vi "TCP Engine Get Msg From Host.vi"(8 "error in (no error)":errorcluster, 11 "Data Cluster in":T1 {"Hardware Info"."Is Present?" items=["Initializing"=-2, "Unknown"=-1, "Not Present"=0, "Present"=1]}) -> (0 "error out":errorcluster, 3 "Data Cluster out":T1 {"Hardware Info"."Is Present?" items=["Initializing"=-2, "Unknown"=-1, "Not Present"=0, "Present"=1]})   [LabVIEW 2024, in "TCP Engine.lvlib"]
uses:
  TCP Engine.lvlib
  Controls/TCP Engine State Machine Data Cluster.ctl
  Controls/TCP Engine Send Loop Data.ctl
  Main Engine/Controls/Main Engine Command Cluster.ctl
  Main Engine/Controls/Main Engine TCP Command Data.ctl
  Main Engine/Controls/Main Engine Hardware Info Data Cluster.ctl
  Controls/TCP Engine Q Driver Options.ctl
  Controls/TCP Engine State Machine Cases.ctl
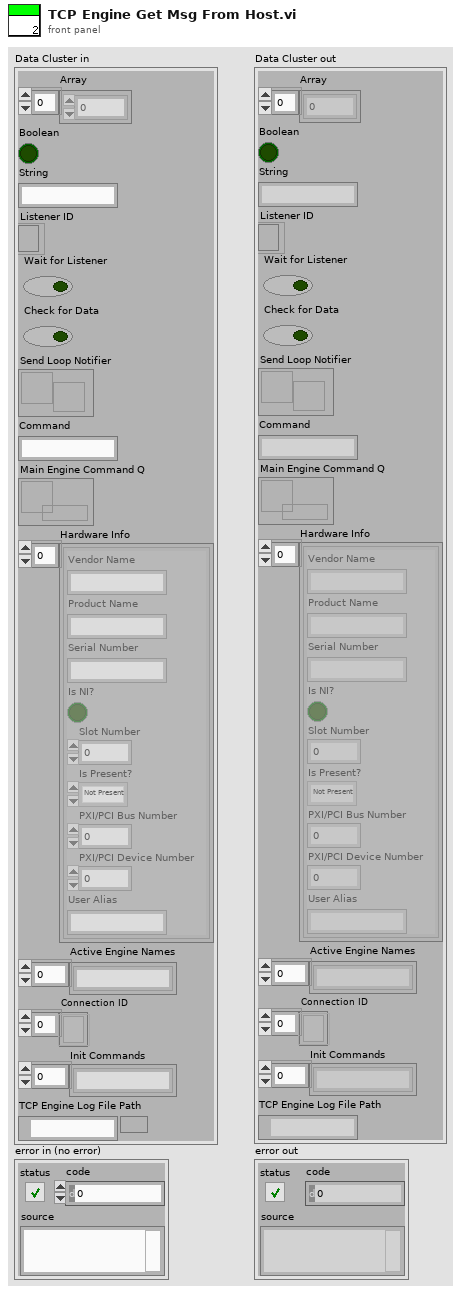
[diagram p1: front panel]
types:
  T1 = typedef "TCP Engine.lvlib/TCP Engine State Machine Data Cluster.ctl" = cluster{"Array":dbl[], "Boolean":bool, "String":string, "Listener ID":refnum<k5>, "Wait for Listener":bool, "Check for Data":bool, "Send Loop Notifier":refnum<notifier>, "Command":string, "Main Engine Command Q":refnum<queue>, "Hardware Info":T2[], "Active Engine Names":string[], "Connection ID":refnum<k5>[], "Init Commands":string[], "TCP Engine Log File Path":path}
  T2 = typedef "Main Engine Hardware Info Data Cluster.ctl" = cluster{"Vendor Name":string, "Product Name":string, "Serial Number":string, "Is NI?":bool, "Slot Number":i32, "Is Present?":i32, "PXI/PCI Bus Number":u32, "PXI/PCI Device Number":u32, "User Alias":string}
  T3 = enum16{"Standard", "Buffered", "CRLF", "Immediate"}
  T4 = typedef "TCP Engine.lvlib/TCP Engine Q Driver Options.ctl" = enum16{"Initialize", "EnQ", "DeQ", "EnQ at Opp", "Get Q Status", "Flush Q", "Release Q"}
  T5 = enum16{"big-endian, network order", "native, host order", "little-endian"}
  T6 = typedef "TCP Engine.lvlib/TCP Engine State Machine Cases.ctl" = enum16{">Poll", ".........State Machine.........", ">Init", ">Init Configuration", ">Decode Configuration", ">Error", ">Exit", "..........TCP Engine..........", ">Wait for Listener", ">Get Msg from HOST", ">Decode the Command", ">Create Listerner ID"}
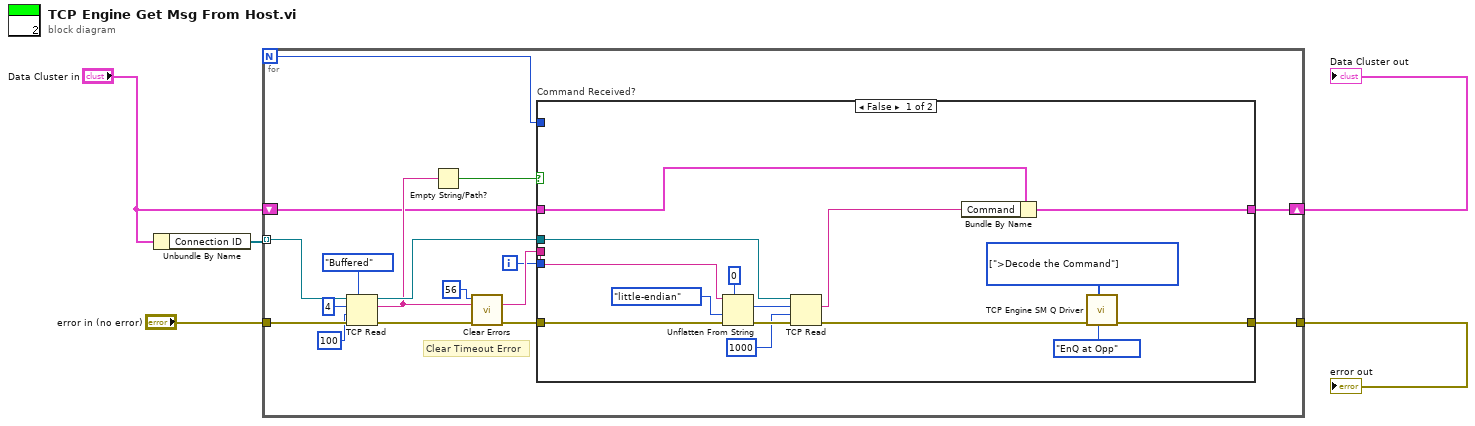
[diagram p0: block diagram]
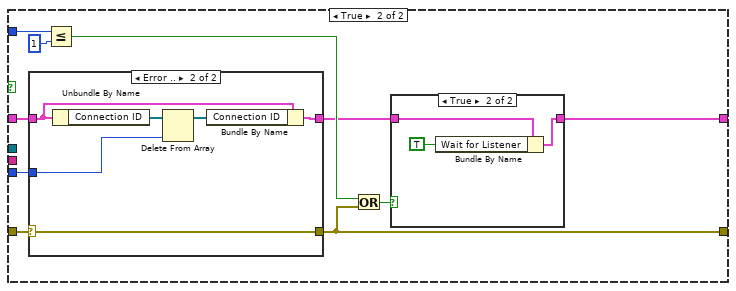
[diagram p2: hidden frame]
diagram:
  n1 = Unbundle By Name("Data Cluster in") -> ("Connection ID"=w1:refnum<k5>[])
  n2 = for {
    N -> [w8]
    tunnel: w1 -> [w21] mode=indexing
    tunnel: "error in (no error)" -> [w20]
    tunnel: [w9] -> w5
    shift-right: [w11] -> w4
    shift-left: "Data Cluster in" -> [w7]
    i -> [w6]
    # "Clear Timeout Error"
    n3 = TCP Read(connection ID=w21, bytes to read=4, error in (no error)=w20, 7:T3."Buffered" ("mode (standard)"), 9:100 ("timeout ms (25000)")) -> (connection ID out=w13:refnum<k5>, data out=w12:string, error out=w16:errorcluster)
    n4 = Empty String/Path?(string/path=w12) -> (empty?=w14:bool)
    n5 = call <vilib>:"Clear Errors.vi"("error in (no error)"=w16, "specific error code to clear (0: all)"=56) -> ("error out"=w10:errorcluster)  [unwired: 4 in, 1 out]
    n6 = case "Command Received?" shown="False" w14 {
      tunnel: w13 -> [w31 _]
      tunnel: w12 -> [w36 _]
      tunnel: w10 -> [w33 w42]
      tunnel: [w28 w46] -> w11
      tunnel: [w25 w37] -> w9
      tunnel: w8 -> [_ w45]
      tunnel: w7 -> [w23 w41]
      tunnel: w6 -> [_ w40]
      frame False {
        w24 = T6[] [enum.">Decode the Command"] items=[">Poll", ".........State Machine.........", ">Init", ">Init Configuration", ">Decode Configuration", ">Error", ">Exit", "..........TCP Engine..........", ">Wait for Listener", ">Get Msg from HOST", ">Decode the Command", ">Create Listerner ID"] ("States")
        n7 = Unflatten From String(type=0 ("length"), binary string=w36, byte order (0:big-endian, network order)=T5."little-endian", error in (no error)=w33) -> (value=w32:i32, error out=w30:errorcluster)  [unwired: 1 in, 1 out]
        n8 = TCP Read(connection ID=w31, bytes to read=w32, error in (no error)=w30, 9:1000 ("timeout ms (25000)")) -> (data out=w22:string, error out=w26:errorcluster)  [unwired: 1 in, 1 out]
        n9 = Bundle By Name(cluster=w23, "Command"=w22) -> (w28:T1)
        n10 = call "TCP Engine SM Q Driver.vi"("Q Driver Options"=TCP_Engine_Q_Driver_Options."EnQ at Opp", "States"=w24, "error in"=w26) -> ("error out"=w25:errorcluster)  [unwired: 4 in, 4 out]
      }
      frame True {
        n11 = case shown="Error .." w42 {
          selector: w42 -> [w47 w49]
          tunnel: w41 -> [w48 w52]
          tunnel: w40 -> [_ w53]
          tunnel: [w48 w50] -> w39
          tunnel: [w47 w49] -> w37
          frame No Error {
          }
          frame Error {
            n12 = Unbundle By Name(w52) -> ("Connection ID"=w54:refnum<k5>[])
            n13 = Delete From Array(array=w54, index=w53) -> (array with subset deleted=w51:refnum<k5>[])  [unwired: 1 in, 1 out]
            n14 = Bundle By Name(cluster=w52, "Connection ID"=w51) -> (w50:T1)
          }
        }
        n15 = Less Or Equal?(x=w45, y=1) -> (x <= y?=w43:bool)
        n16 = Or(x=w43, y=w37) -> (x .or. y?=w38:bool)
        n17 = case shown="True" w38 {
          tunnel: w39 -> [w55 w58]
          tunnel: [w55 w57] -> w46
          frame False {
          }
          frame True {
            n18 = Bundle By Name(cluster=w58, "Wait for Listener"=TRUE) -> (w57:T1)
          }
        }
      }
    }
  }
  "error out" <- w5
  "Data Cluster out" <- w4
